vi "Define 1D Wave PDE (VIRef).vi"(0 "PDE in":refnum<class "NI_PDE.lvclass">, 1 "data":variant, 5 "F(t, x)":refnum<vi>, 7 "k":dbl=1.0, 9 "a":dbl, 11 "error in (no error)":errorcluster) -> (4 "PDE out":refnum<class "NI_PDE.lvclass">, 15 "error out":errorcluster)   [LabVIEW 2020, in "NI_PDE.lvlib"]
doc: "Defines the right side of a partial differential equation and its coefficients. You must manually select the polymorphic instance to use."
uses:
  <vilib>/gmath/NI_PDE.lvlib
  <vilib>/gmath/pde.llb/PDEClass/NI_PDE.lvclass
  <vilib>/gmath/pde.llb/RHSClass/RHS_2D_VIRef/NI_RHS_2D_VIRef.lvclass
  e:/builds/penguin/labview/branches/2020/dev/dist/vi.lib/gmath/pde.llb/RHSClass/NI_RHS.lvclass
  <vilib>/gmath/pde.llb/PDEClass/PDE_Wave_1D/NI_PDE_Wave_1D.lvclass
  e:/builds/penguin/labview/branches/2020/dev/dist/vi.lib/gmath/pde.llb/PDEClass/NI_PDE.lvclass
  <vilib>/gmath/pde.llb/PDEClass/PDE_2ndOrder_ConstPara/Para Data.ctl
  <vilib>/gmath/pde.llb/RHSClass/RHS_2D_VIRef/RHS Data.ctl
  <vilib>/gmath/pde.llb/PDEClass/PDE_2ndOrder_ConstPara/NI_PDE_2ndOrder_ConstPara.lvclass
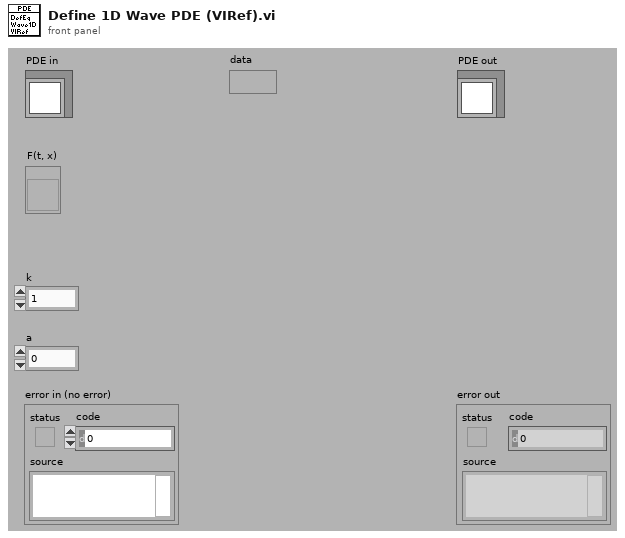
[diagram p1: front panel]
types:
  T1 = typedef "NI_PDE.lvlib/NI_RHS_2D_VIRef.lvclass/RHS Data.ctl" = cluster{"F":refnum<vi>, "data":variant}
  T2 = typedef "NI_PDE.lvlib/NI_PDE_2ndOrder_ConstPara.lvclass/Para Data.ctl" = cluster{"k":dbl, "a":dbl}
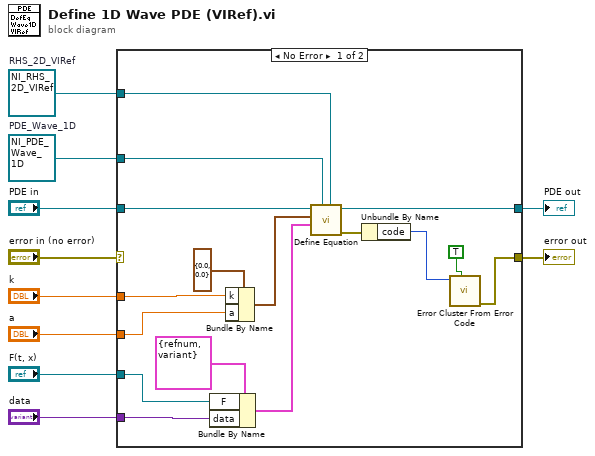
[diagram p0: block diagram]
diagram:
  w1 = refnum<class "NI_PDE_Wave_1D.lvclass"> refnum  # PDE_Wave_1D
  w2 = refnum<class "NI_RHS_2D_VIRef.lvclass"> refnum  # RHS_2D_VIRef
  n1 = case shown="No Error" "error in (no error)" {
    selector: "error in (no error)" -> [_ w28]
    tunnel: "PDE in" -> [w13 w27]
    tunnel: [w19 w27] -> w9
    tunnel: "F(t, x)" -> [w15 _]
    tunnel: "a" -> [w16 _]
    tunnel: "k" -> [w17 _]
    tunnel: "data" -> [w14 _]
    tunnel: [w24 w28] -> w4
    tunnel: w2 -> [w12 _]
    tunnel: w1 -> [w11 _]
    frame No Error {
      n2 = Bundle By Name(cluster=T1 {"F"=refnum, "data"=variant} ("RHS data"), "F"=w15, "data"=w14) -> (w20:T1)
      n3 = Bundle By Name(cluster=T2 {"k"=0.0, "a"=0.0} ("para data"), "k"=w17, "a"=w16) -> (w21:T2)
      n4 = call <vilib>:"Define Equation.vi"("target RHS"=w12, "target PDE"=w11, "RHS"=w20, "parameter"=w21, "PDE in"=w13) -> ("error out"=w18:errorcluster, "PDE out"=w19:refnum<class "NI_PDE.lvclass">)  [unwired: 1 in, 4 out]
      n5 = Unbundle By Name(w18) -> ("code"=w26:i32)
      n6 = call <vilib>:"Error Cluster From Error Code.vi"("show call chain? (False)"=TRUE, "error code (0)"=w26) -> ("error out"=w24:errorcluster)  [unwired: 1 in, 6 out]
    }
    frame Error {
    }
  }
  "PDE out" <- w9
  "error out" <- w4
